vi "TGood.vi"() -> ()   [LabVIEW 2014]
uses:
  ESLSCDLL.dll
panel:
  out "Boolesch":bool
  in  "channel 1 or 2":u32=1
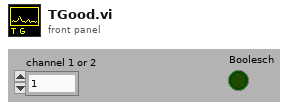
[diagram p1: front panel]
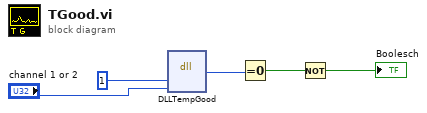
[diagram p0: block diagram]
diagram:
  n1 = dll-call lib="C:/Users/Gerhard/Documents/New64/lv/1cam/board.vis/ESLSCDLL.dll" fn="DLLTempGood"("drv"=u32 1, "ch"="channel 1 or 2") -> ("Rückgabetyp"=w3:u8)  [unwired: 5 in, 2 out]
  n2 = Equal To 0?(x=w3) -> (x = 0?=w2:bool)
  n3 = Not(x=w2) -> (.not. x?=→"Boolesch":bool)
